vi "Get Dependency.vi"(8 "error in (no error)":errorcluster, 11 "object in":refnum<class "DAQ.lvclass">) -> (0 "error out":errorcluster, 2 "Dependency":T1, 3 "object out":refnum<class "DAQ.lvclass">)   [LabVIEW 2022 SP3, in "DAQ.lvclass"]
doc: "Developed by Kevin Thompson\nkevin@thompsonengineering.net\n\nCopyright 2018-2020\nThompson Engineering, LLC"
uses:
  DAQ.lvclass
  DAQ.lvclass/DAQ.ctl
  Support/DataQueues/DataQueues.lvclass
  DataTypes/Dependency--cluster.ctl
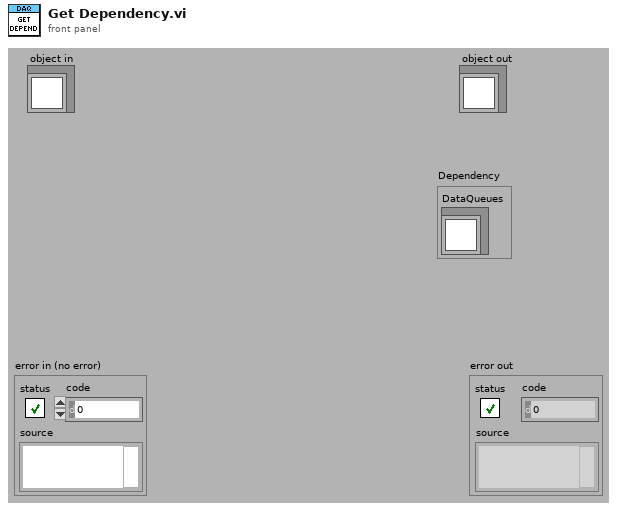
[diagram p1: front panel]
types:
  T1 = typedef "DAQ.lvclass/Dependency--cluster.ctl" = cluster{"DataQueues":refnum<class "DataQueues.lvclass">}
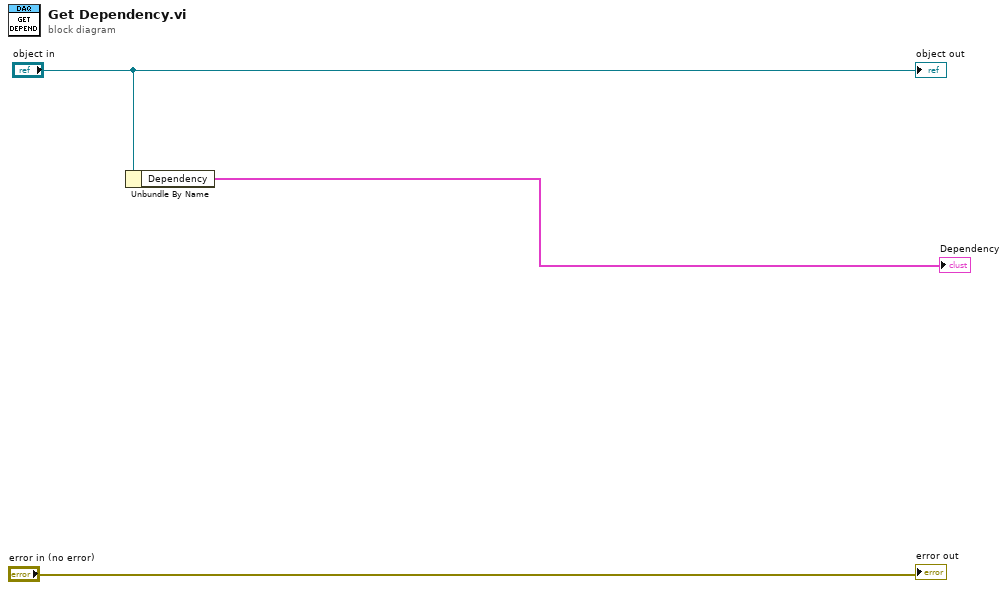
[diagram p0: block diagram]
diagram:
  n1 = Unbundle By Name("object in") -> ("Dependency"=→"Dependency":T1)
  "error out" <- "error in (no error)"
  "object out" <- "object in"
